vi "Close PDFStamper.vi"(0 "PDFStamper":refnum<k24>, 11 "error in (no error)":errorcluster) -> (15 "error out":errorcluster)   [LabVIEW 2012]
doc: "Developed by Jean-Marc Simard\nCopyright © 2010, Exaprom Inc.\nAll rights reserved.\nLicense: BSD\n\nWith iTextSharp 4.1.6 (http://itextsharp.sourceforge.net)\nunder Mozilla Public License Version 1.1\n(http://www.mozilla.org/MPL/MPL-1.1.html)"
uses:
  C:/Users/MaxCorp/Documents/TopPerm - Base/DLL/itextsharp.dll
  DLL/itextsharp.dll
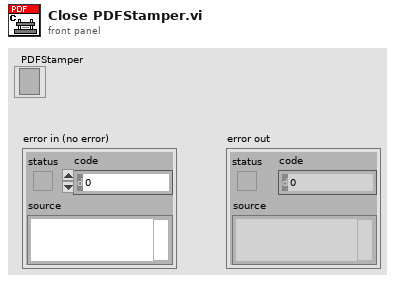
[diagram p1: front panel]
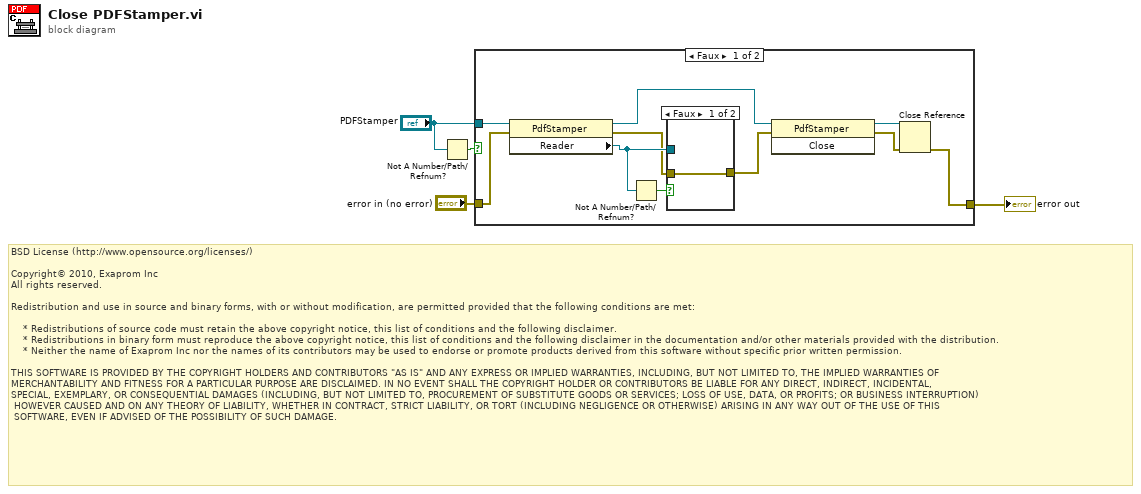
[diagram p0: block diagram]
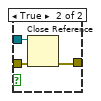
[diagram p2: hidden frame]
diagram:
  # "BSD License (http://www.opensource.org/licenses/)\n\nCopyright© 2010, Exaprom Inc\nAll rights reserved.\n\nRedistribution and use in source and binary forms, with or without modification, are permitted provided that the following conditions are met:\n\n    * Redistributions of source code must retain the above copyright notice, this list of conditions and the following disclaimer.\n    * Redistributions in binary form must reproduce the above copyright notice, this list of conditions and the following disclaimer in the documentation and/or other materials provided with the distribution.\n    * Neither the name of Exaprom Inc nor the names of its contributors may be used to endorse or promote products derived from this software without specific prior written permission.\n\nTHIS SOFTWARE IS PROVIDED BY THE COPYRIGHT HOLDERS AND CONTRIBUTORS \"AS IS\" AND ANY EXPRESS OR IMPLIED WARRANTIES, INCLUDING, BUT NOT LIMITED TO, THE IMPLIED WARRANTIES OF \nMERCHANTABILITY AND FITNESS FOR A PARTICULAR PURPOSE ARE DISCLAIMED. IN NO EVENT SHALL THE COPYRIGHT HOLDER OR CONTRIBUTORS BE LIABLE FOR ANY DIRECT, INDIRECT, INCIDENTAL,\nSPECIAL, EXEMPLARY, OR CONSEQUENTIAL DAMAGES (INCLUDING, BUT NOT LIMITED TO, PROCUREMENT OF SUBSTITUTE GOODS OR SERVICES; LOSS OF USE, DATA, OR PROFITS; OR BUSINESS INTERRUPTION)\n HOWEVER CAUSED AND ON ANY THEORY OF LIABILITY, WHETHER IN CONTRACT, STRICT LIABILITY, OR TORT (INCLUDING NEGLIGENCE OR OTHERWISE) ARISING IN ANY WAY OUT OF THE USE OF THIS\n SOFTWARE, EVEN IF ADVISED OF THE POSSIBILITY OF SUCH DAMAGE."
  n1 = Not A Number/Path/Refnum?(number/path/refnum="PDFStamper") -> (NaN/Path/Refnum?=w3:bool)
  n2 = case shown="Faux" w3 {
    tunnel: [w11 w19] -> w4
    tunnel: "PDFStamper" -> [w10 _]
    tunnel: "error in (no error)" -> [w5 w19]
    frame False {
      n3 = property class="PdfStamper"(reference=w10, error in=w5) -> (reference out=w14:refnum<k24>, error out=w7:errorcluster, "Reader"=w9:refnum<k24>)
      n4 = Not A Number/Path/Refnum?(number/path/refnum=w9) -> (NaN/Path/Refnum?=w8:bool)
      n5 = case shown="Faux" w8 {
        tunnel: w9 -> [_ w18]
        tunnel: w7 -> [w15 w17]
        tunnel: [w15 w16] -> w6
        frame False {
        }
        frame True {
          n6 = Close Reference(reference=w18, error in (no error)=w17) -> (error out=w16:errorcluster)
        }
      }
      n7 = invoke class="PdfStamper" method="Close"(reference=w14, error in=w6) -> (reference out=w12:refnum<k24>, error out=w13:errorcluster)  [unwired: 1 in, 1 out]
      n8 = Close Reference(reference=w12, error in (no error)=w13) -> (error out=w11:errorcluster)
    }
    frame True {
    }
  }
  "error out" <- w4
